vi "数组至字符逗号隔开转化.vi"(11 "数组data in":string[](array[string])) -> (3 "逗号隔开出":string)   [LabVIEW 2017]
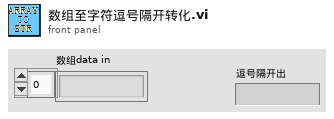
[diagram p1: front panel]
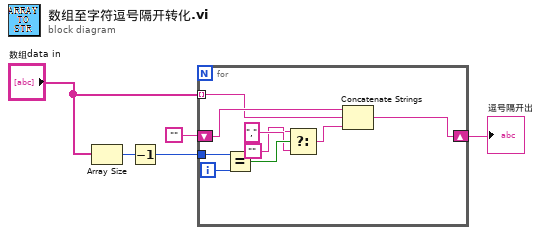
[diagram p0: block diagram]
diagram:
  n1 = Array Size(array="数组data in") -> (size(s)=w4:i32)
  n2 = Decrement(x=w4) -> (x-1=w3:i32)
  n3 = for {
    tunnel: "数组data in" -> [w13] mode=indexing
    shift-right: [w6] -> w1
    shift-left: "" -> [w14]
    tunnel: w3 -> [w12]
    i -> [w11]
    n4 = Equal?(x=w12, y=w11) -> (x = y?=w10:bool)
    n5 = Select(t="", s=w10, f=",") -> (s? t:f=w7:string)
    n6 = Concatenate Strings(w14, w13, w7) -> (w6:string)
  }
  "逗号隔开出" <- w1
